vi "Add Monitoring port tree.vi"(8 "Error In":errorcluster, 10 "NI-XNET Port (Item Ref)":T1 format="%.0x", 11 "Device Item Ref in":T1 format="%.0x") -> (0 "Error Out":errorcluster, 3 "Device Item Ref Out":T1 format="%.0x")   [LabVIEW 2018, in "NI-XNET Monitor System Explorer.lvlib"]
uses:
  NI-XNET Monitor System Explorer.lvlib
  <vilib>/NI Veristand/Custom Device API/Custom Device Item Ref.ctl
  <vilib>/NI Veristand/Custom Device Tools/Custom Device Utility Library/Search Direction.ctl
  Shared/Constants.vi
  <vilib>/NI Veristand/Custom Device Tools/Custom Device Utility Library/NI VeriStand - Search for Item by GUID.vi
  <vilib>/NI Veristand/Custom Device API/Set Item Property (String).vi
  <vilib>/NI Veristand/Custom Device API/Set Item Property (Boolean).vi
  <vilib>/NI Veristand/Custom Device API/Custom Device API.lvlib
  Shared/NI-XNET Monitor Shared.lvlib
  <vilib>/NI Veristand/Custom Device Tools/Custom Device Utility Library/Custom Device Utility Library.lvlib
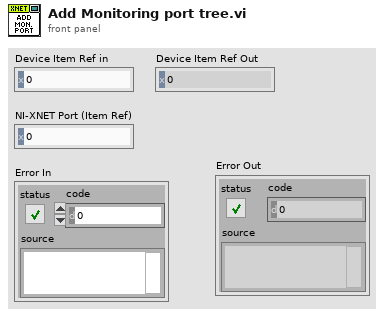
[diagram p1: front panel]
types:
  T1 = typedef "Custom Device API.lvlib/Custom Device Item Ref.ctl" = u64
  T2 = typedef "Custom Device API.lvlib/Custom Device Item Info.ctl" = cluster{"Name":string, "Is Channel":bool, "GUID":string, "Is Waveform":bool}
  T3 = typedef "Custom Device Utility Library.lvlib/Search Direction.ctl" = enum16{"Down", "Up"}
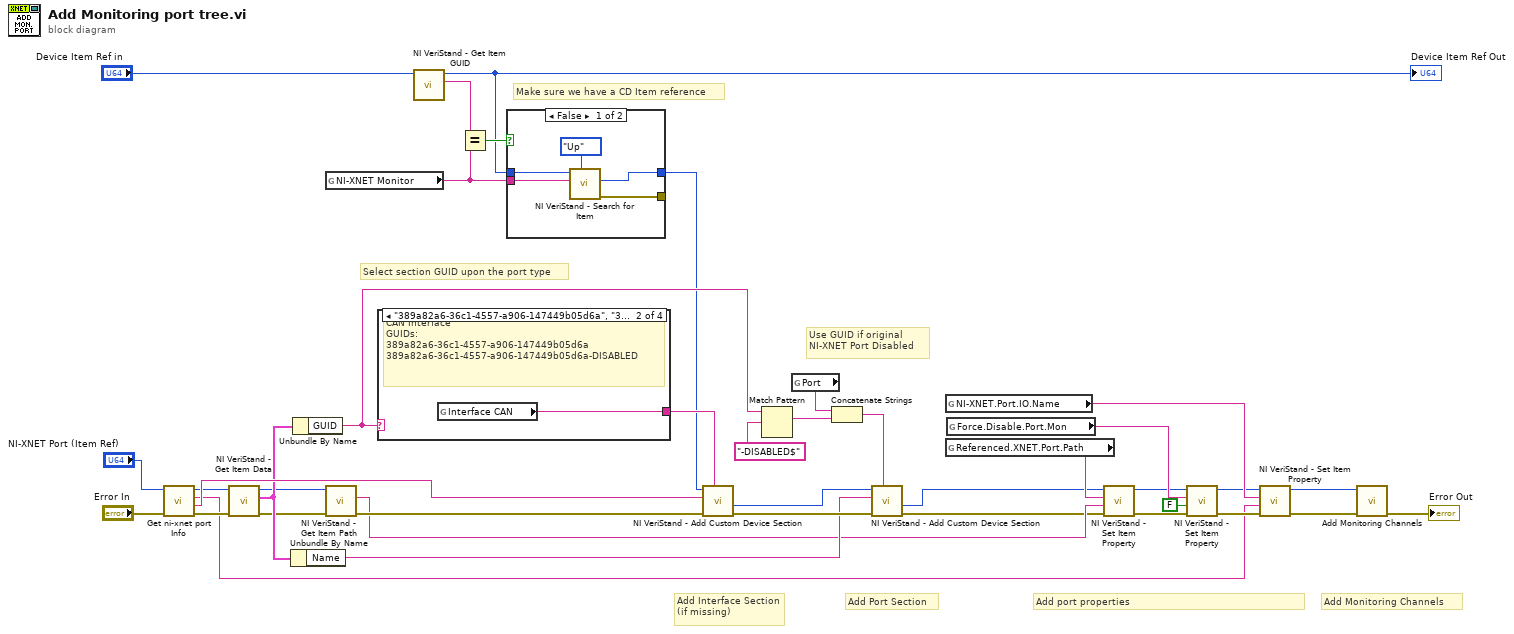
[diagram p0: block diagram]
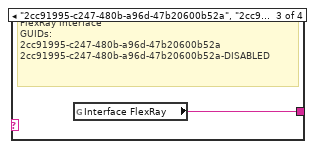
[diagram p4: hidden frame]
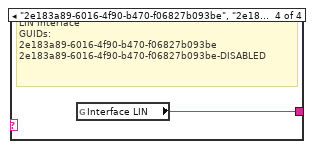
[diagram p5: hidden frame]
diagram:
  # "Make sure we have a CD Item reference"
  # "Add Monitoring Channels"
  # "Add port properties"
  # "Select section GUID upon the port type"
  # "Use GUID if original\nNI-XNET Port Disabled"
  # "Add Port Section"
  # "Add Interface Section (if missing)"
  n1 = call "Get ni-xnet port Info.vi"("Error In"="Error In", "NI-XNET Port Item Ref in"="NI-XNET Port (Item Ref)") -> ("Error Out"=w15:errorcluster, "NI-XNET Port Type"=w30:string, "NI-XNET Port Name"=w14:string, "NI-XNET Port Item Ref out"=w16:T1)  [unwired: 5 in, 1 out]
  n2 = call <vilib>:"NI VeriStand - Get Item Data.vi"("error in (no error)"=w15, "Item Ref in"=w16) -> ("error out"=w5:errorcluster, "Item Info"=w25:T2, "Item Ref out"=w7:T1)  [unwired: 6 in, 1 out]
  n3 = Unbundle By Name(w25) -> ("Name"=w24:string)
  n4 = Unbundle By Name(w25) -> ("GUID"=w26:string)
  n5 = global read "Constants.vi" "NI-XNET Monitor"() -> (w12:string)
  n6 = call <vilib>:"NI VeriStand - Get Item Path.vi"("error in (no error)"=w5, "Item Ref in"=w7) -> ("error out"=w6:errorcluster, "Path"=w4:string)  [unwired: 6 in, 2 out]
  n7 = case shown="\"389a82a6-36c1-4557-a906-147449b05d6a\", \"389a82a6-36c1-4557-a906-147449b05d6a-DISABLED\"" w26 {
    tunnel: [_ w40 w41 w42] -> w34
    frame Default {
    }
    frame "389a82a6-36c1-4557-a906-147449b05d6a", "389a82a6-36c1-4557-a906-147449b05d6a-DISABLED" {
      # "CAN Interface\nGUIDs:\n389a82a6-36c1-4557-a906-147449b05d6a\n389a82a6-36c1-4557-a906-147449b05d6a-DISABLED"
      n8 = global read "Constants.vi" "Interface CAN"() -> (w40:string)
    }
    frame "2cc91995-c247-480b-a96d-47b20600b52a", "2cc91995-c247-480b-a96d-47b20600b52a-DISABLED" {
      # "FlexRay Interface\nGUIDs:\n2cc91995-c247-480b-a96d-47b20600b52a\n2cc91995-c247-480b-a96d-47b20600b52a-DISABLED"
      n9 = global read "Constants.vi" "Interface FlexRay"() -> (w41:string)
    }
    frame "2e183a89-6016-4f90-b470-f06827b093be", "2e183a89-6016-4f90-b470-f06827b093be-DISABLED" {
      # "LIN Interface\nGUIDs:\n2e183a89-6016-4f90-b470-f06827b093be\n2e183a89-6016-4f90-b470-f06827b093be-DISABLED"
      n10 = global read "Constants.vi" "Interface LIN"() -> (w42:string)
    }
  }
  n11 = call <vilib>:"NI VeriStand - Get Item GUID.vi"("Item Ref in"="Device Item Ref in") -> ("GUID"=w13:string, "Item Ref out"=w8:T1)  [unwired: 8 in, 1 out]
  "Device Item Ref Out" <- w8
  n12 = Equal?(x=w13, y=w12) -> (x = y?=w11:bool)
  n13 = case shown="False" w11 {
    tunnel: [w46 _] -> _
    tunnel: [w45 w48] -> w10
    tunnel: w8 -> [w44 w48]
    tunnel: w12 -> [w43 _]
    frame False {
      n14 = call-poly <vilib>:"NI VeriStand - Search for Item.vi"("Direction (Down)"=Search_Direction."Up", "Item GUID"=w43, "Section Ref in"=w44) -> ("error out"=w46:errorcluster, "Item Ref"=w45:T1)  [unwired: 5 in, 2 out]
    }
    frame True {
    }
  }
  n15 = call <vilib>:"NI VeriStand - Add Custom Device Section.vi"("GUID (Default Section)"=w34, "error in (no error)"=w6, "Section Name"=w30, "Parent Ref in"=w10) -> ("error out"=w27:errorcluster, "Section Ptr"=w31:T1)  [unwired: 4 in, 2 out]
  n16 = Match Pattern(string=w26, regular expression="-DISABLED$") -> (match substring=w28:string)  [unwired: 1 in, 3 out]
  n17 = global read "Constants.vi" "Port"() -> (w32:string)
  n18 = Concatenate Strings(w32, w28) -> (w33:string)
  n19 = call <vilib>:"NI VeriStand - Add Custom Device Section.vi"("GUID (Default Section)"=w33, "error in (no error)"=w27, "Section Name"=w24, "Parent Ref in"=w31) -> ("error out"=w3:errorcluster, "Section Ptr"=w2:T1)  [unwired: 4 in, 2 out]
  n20 = global read "Constants.vi" "NI-XNET.Port.IO.Name"() -> (w22:string)
  n21 = global read "Constants.vi" "Referenced.XNET.Port.Path"() -> (w35:string)
  n22 = global read "Constants.vi" "Force.Disable.Port.Mon"() -> (w38:string)
  n23 = call-poly <vilib>:"NI VeriStand - Set Item Property.vi"("error in (no error)"=w3, "Value"=w4, "Property Name"=w35, "Item Ref in"=w2) -> ("error out"=w36:errorcluster, "Item Ref out"=w37:T1)  [unwired: 5 in, 1 out]
  n24 = call-poly <vilib>:"NI VeriStand - Set Item Property.vi"("error in (no error)"=w36, "Value"=FALSE, "Property Name"=w38, "Item Ref in"=w37) -> ("error out"=w18:errorcluster, "Item Ref out"=w21:T1)  [unwired: 5 in, 1 out]
  n25 = call-poly <vilib>:"NI VeriStand - Set Item Property.vi"("error in (no error)"=w18, "Value"=w14, "Property Name"=w22, "Item Ref in"=w21) -> ("error out"=w19:errorcluster, "Item Ref out"=w20:T1)  [unwired: 5 in, 1 out]
  n26 = call "Add Monitoring Channels.vi"("Error In"=w19, "Port Section Item Ref in"=w20) -> ("Error Out"=→"Error Out":errorcluster)  [unwired: 8 in, 1 out]
